vi "VisionRect.vi"(0 "Image In":T2, 1 "Red BCG Values (Brightness 1)":T1={"Brightness"=82.739365, "Contrast"=81.04256, "Gamma"=10.0}, 2 "Green BCG Values (Brightness 1)":T1={"Brightness"=82.739365, "Contrast"=81.04256, "Gamma"=10.0}, 3 "Blue BCG Values (Brightness 1)":T1={"Brightness"=82.739365, "Contrast"=81.04256, "Gamma"=10.0}, 7 "error in":errorcluster) -> (20 "Image Out":T2, 27 "error out":errorcluster)   [LabVIEW 2020]
uses:
  <vilib>/vision/Image Controls.llb/IMAQ Image.ctl
  <vilib>/vision/NI_Vision_Development_Module.lvlib
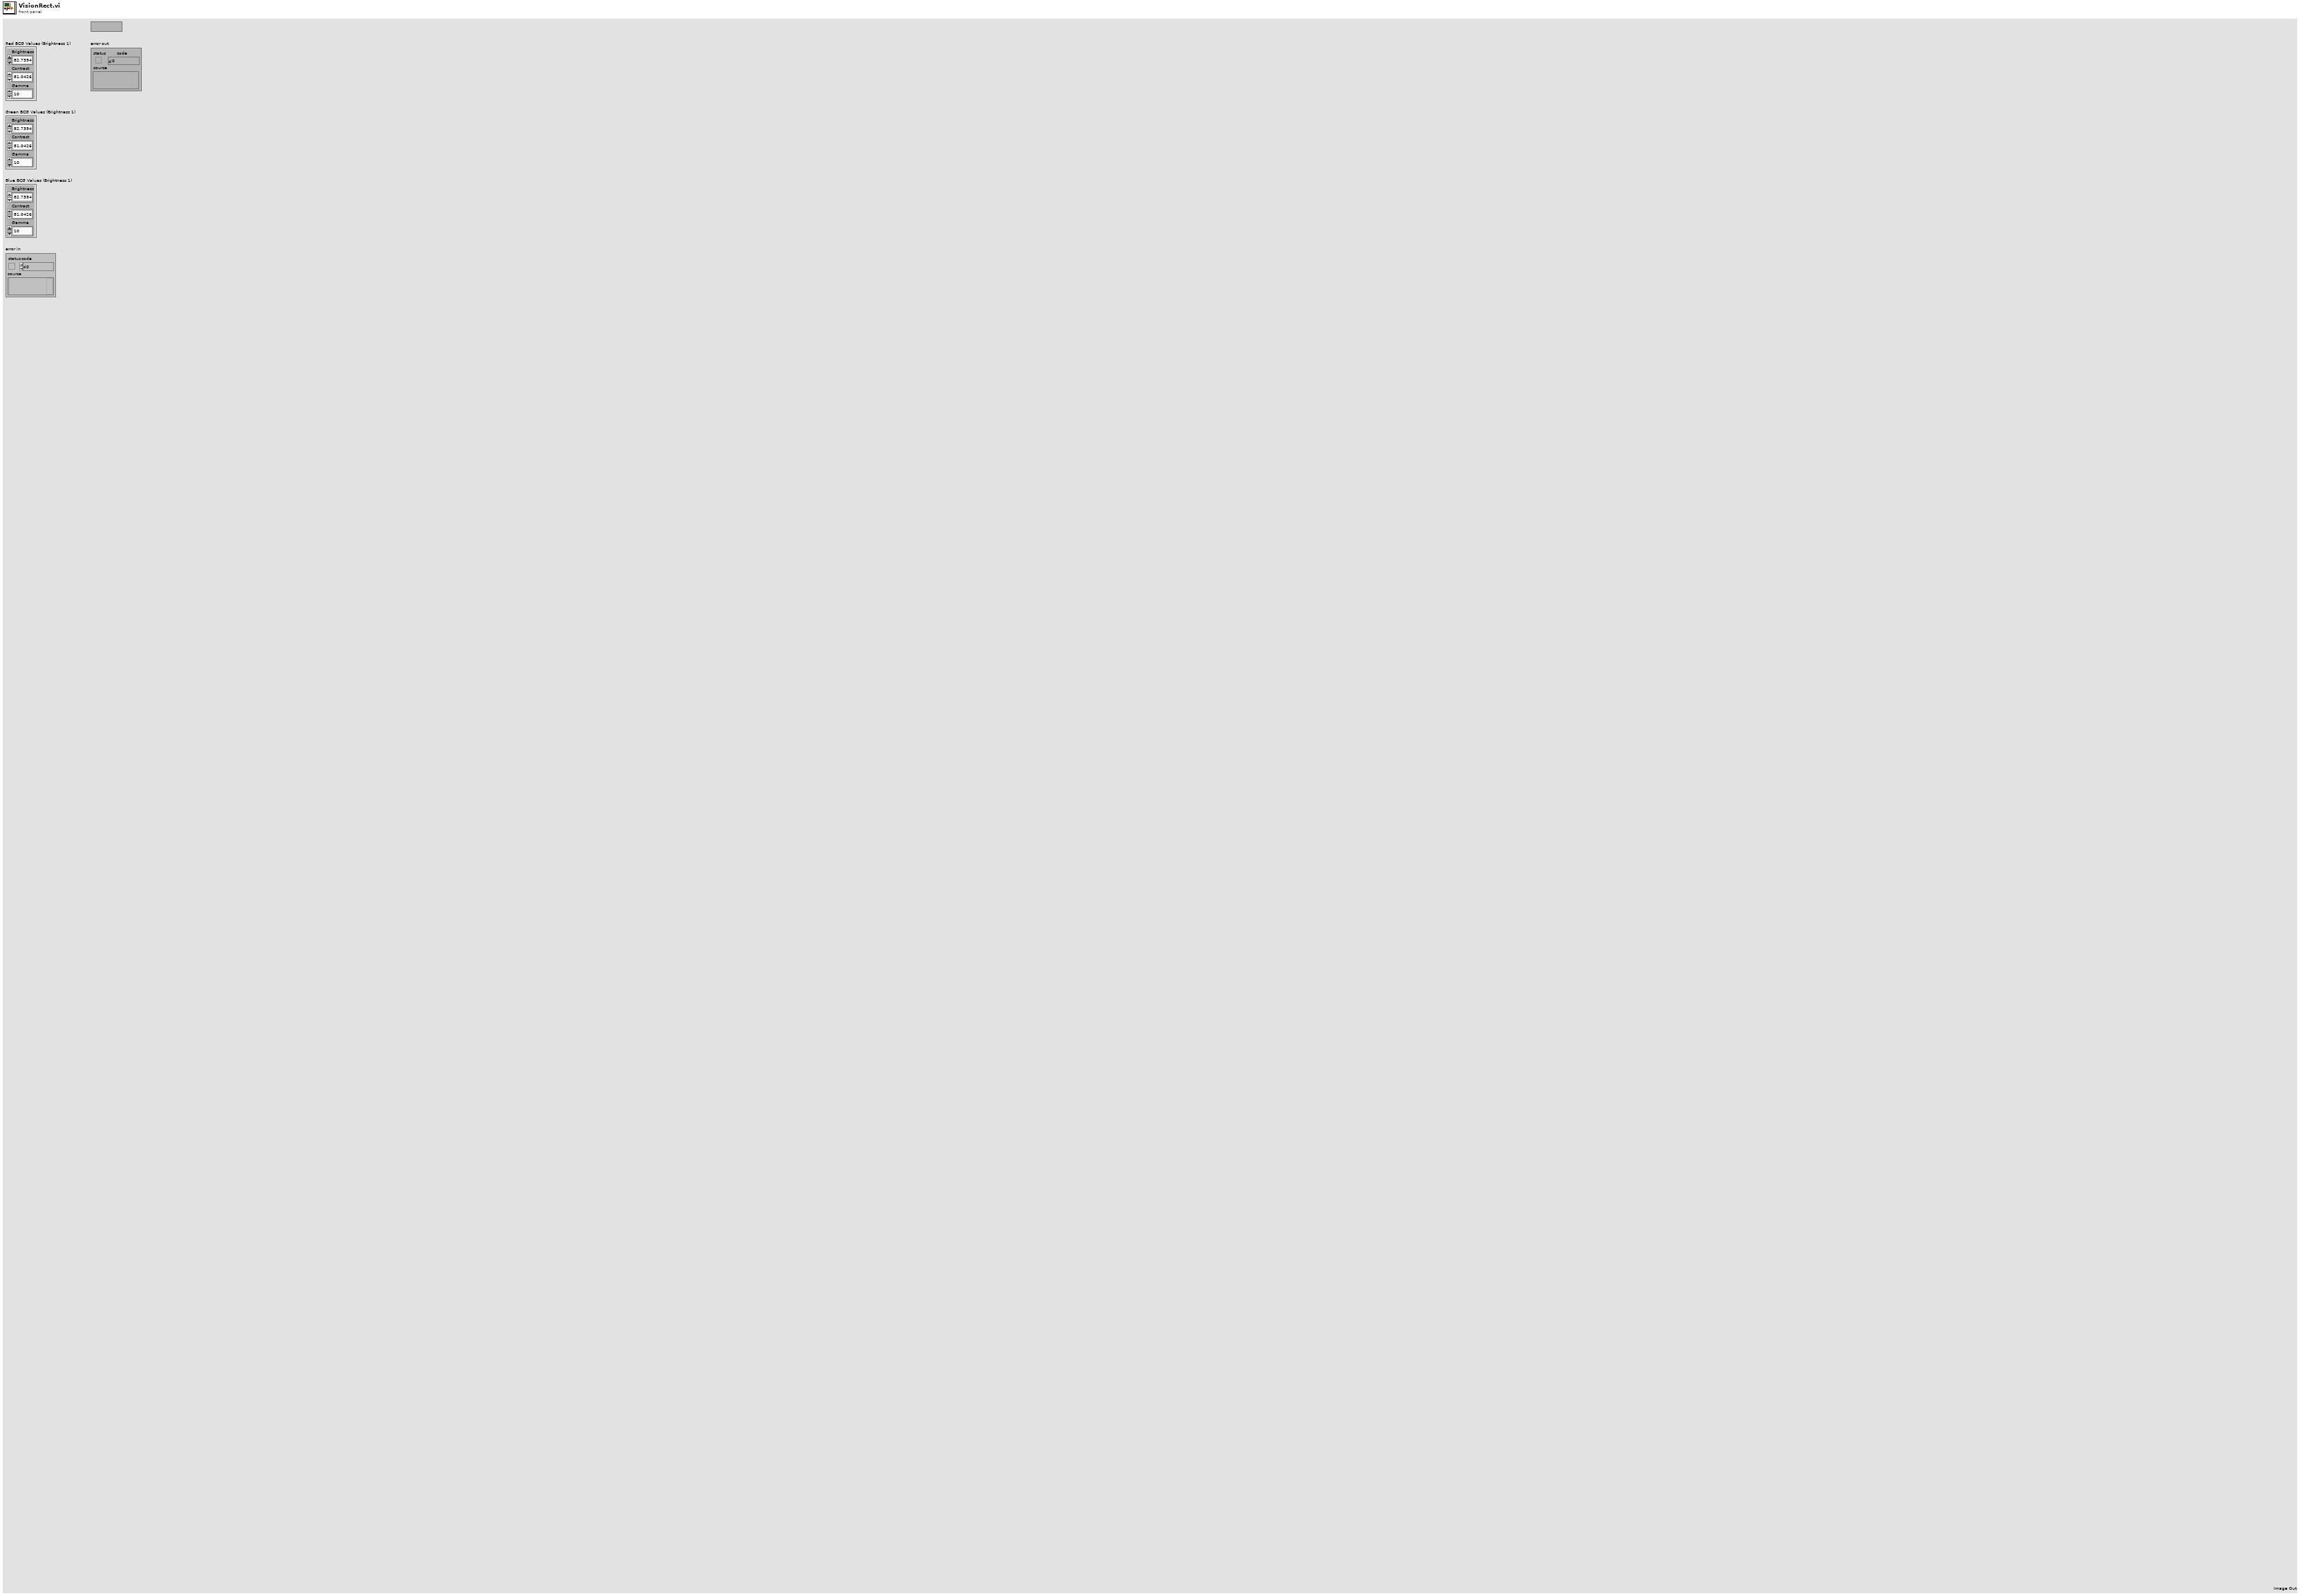
[diagram p1: front panel]
types:
  T1 = cluster{"Brightness":sgl, "Contrast":sgl, "Gamma":sgl}
  T2 = typedef "IMAQ Image.ctl" = refnum<image>
  T3 = cluster{"Measurement Parameter":i32, "Range Lower Value":dbl, "Range Upper Value":dbl, "Range":bool, "Measurement Type":bool}[]
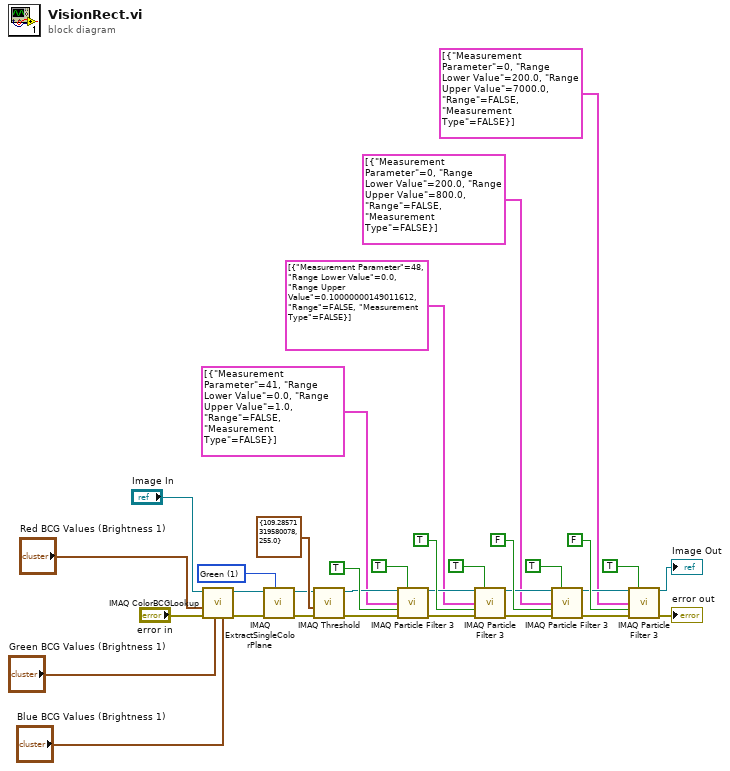
[diagram p0: block diagram]
diagram:
  w28 = 1 items=["Red", "Green", "Blue", "Hue", "Saturation", "Luminance", "Value", "Intensity"] ("Color Plane")
  n1 = call "IMAQ ColorBCGLookup"("Blue BCG Values"="Blue BCG Values (Brightness 1)", "Green BCG Values"="Green BCG Values (Brightness 1)", "error in (no error)"="error in", "Red BCG Values"="Red BCG Values (Brightness 1)", "Image Src"="Image In") -> ("error out"=w26:errorcluster, "Image Dst Out"=w27:T2)  [unwired: 2 in, 3 out]
  n2 = call "IMAQ ExtractSingleColorPlane"("Color Plane"=w28, "error in (no error)"=w26, "Image Src"=w27) -> ("error out"=w23:errorcluster, "Image Dst Out"=w24:T2)  [unwired: 1 in, 6 out]
  n3 = call "IMAQ Threshold"("error in (no error)"=w23, "Range"=cluster{"Lower value":sgl, "Upper value":sgl} {"Lower value"=109.28571, "Upper value"=255.0}, "Image Src"=w24) -> ("error out"=w19:errorcluster, "Image Dst Out"=w20:T2)  [unwired: 3 in, 4 out]
  n4 = call "IMAQ Particle Filter 3"("Image Src"=w20, "Connectivity 4/8 (8)"=TRUE, "Selection Values"=T3 [{"Measurement Parameter"=41, "Range Lower Value"=0.0, "Range Upper Value"=1.0, "Range"=FALSE, "Measurement Type"=FALSE}], "Keep/Remove Particles (F)"=TRUE ("Keep/Remove Particles"), "error in (no error)"=w19) -> ("Image Dst Out"=w15:T2, "error out"=w14:errorcluster)  [unwired: 4 in, 5 out]
  n5 = call "IMAQ Particle Filter 3"("Image Src"=w15, "Connectivity 4/8 (8)"=TRUE, "Selection Values"=T3 [{"Measurement Parameter"=48, "Range Lower Value"=0.0, "Range Upper Value"=0.10000000149011612, "Range"=FALSE, "Measurement Type"=FALSE}], "Keep/Remove Particles (F)"=TRUE ("Keep/Remove Particles"), "error in (no error)"=w14) -> ("Image Dst Out"=w10:T2, "error out"=w9:errorcluster)  [unwired: 4 in, 5 out]
  n6 = call "IMAQ Particle Filter 3"("Image Src"=w10, "Connectivity 4/8 (8)"=TRUE, "Selection Values"=T3 [{"Measurement Parameter"=0, "Range Lower Value"=200.0, "Range Upper Value"=800.0, "Range"=FALSE, "Measurement Type"=FALSE}], "Keep/Remove Particles (F)"=FALSE ("Keep/Remove Particles"), "error in (no error)"=w9) -> ("Image Dst Out"=w3:T2, "error out"=w2:errorcluster)  [unwired: 4 in, 5 out]
  n7 = call "IMAQ Particle Filter 3"("Image Src"=w3, "Connectivity 4/8 (8)"=TRUE, "Selection Values"=T3 [{"Measurement Parameter"=0, "Range Lower Value"=200.0, "Range Upper Value"=7000.0, "Range"=FALSE, "Measurement Type"=FALSE}], "Keep/Remove Particles (F)"=FALSE ("Keep/Remove Particles"), "error in (no error)"=w2) -> ("Image Dst Out"=→"Image Out":T2, "error out"=→"error out":errorcluster)  [unwired: 4 in, 5 out]
